vi "create channels for testing.vi"() -> (0 "2d names":string[][](array[string]), 1 "1d names":string[](array[string]), 2 "2d channels":refnum<class "Profibus channel.lvclass">[][](array[class]), 3 "1d channels":refnum<class "Profibus channel.lvclass">[](array[class]))   [LabVIEW 2013, in "Profibus Module tests.lvlib"]
uses:
  Profibus Module tests.lvlib
  channel/Profibus channel.lvclass
  <vilib>/NI/Tag Bus Module Framework/channel/channel classification.ctl
  configuration/Profibus Module configuration.lvclass
  <vilib>/NI/Tag Bus/tag/tag descriptor.lvclass/tag descriptor.ctl
  <vilib>/NI/Tag Bus Module Framework/channel/TBM channel.lvclass/TBM channel.ctl
  <vilib>/NI/Tag Bus/tag/write tag name.vi
  <vilib>/NI/Tag Bus/tag/write data type.vi
  <vilib>/NI/Tag Bus Module Framework/channel/Write channel classification.vi
  <vilib>/NI/Tag Bus Module Framework/channel/TBM channel.lvclass
  <vilib>/NI/Configuration Framework/serializable configuration/NISE_CEF_serializable configuration.lvclass
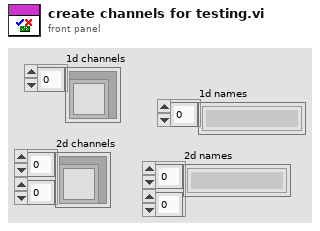
[diagram p1: front panel]
types:
  T1 = typedef "TBM channel.lvclass/channel classification.ctl" = enum16{"input data", "output data", "processing parameter", "processing result"}
  T2 = typedef "tag bus.lvlib/tag descriptor.lvclass/Data Type.ctl" = enum16{"Double", "Single", "I64", "I32", "I16", "I8", "U64", "U32", "U16", "U8", "Boolean", "String", "Array of Double", "Array of Single", "Array of I64", "Array of I32", "Array of I16", "Array of I8", "Array of U64", "Array of U32", "Array of U16", "Array of U8", "Array of Boolean", "Array of String"}
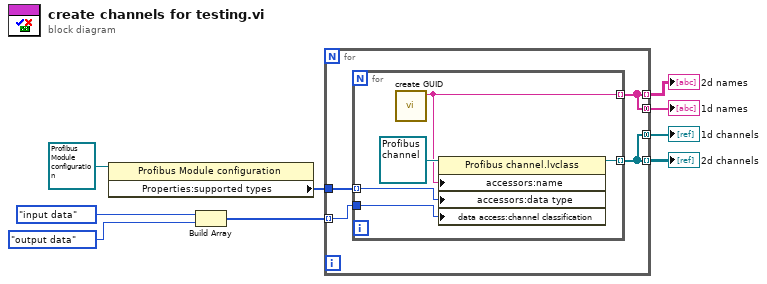
[diagram p0: block diagram]
diagram:
  n1 = property class="Profibus Module configuration"(reference=refnum<class "Profibus Module configuration.lvclass"> refnum ("tag bus configurable plugin module configuration")) -> ("Properties:supported types"=w9:T2[])  [unwired: 1 in, 2 out]
  n2 = Build Array(channel_classification."input data" ("channel classification"), channel_classification."output data" ("channel classification")) -> (w6:T1[])
  n3 = for {
    tunnel: w6 -> [w13] mode=indexing
    tunnel: [w11] -> w7 mode=concatenating
    tunnel: w9 -> [w12]
    tunnel: [w11] -> w3 mode=indexing
    tunnel: [w10] -> w1 mode=concatenating
    tunnel: [w10] -> w2 mode=indexing
    n4 = for {
      tunnel: w13 -> [w15]
      tunnel: [w17] -> w11 mode=indexing
      tunnel: w12 -> [w16] mode=indexing
      tunnel: [w14] -> w10 mode=indexing
      n5 = call <vilib>:"create GUID.vi"() -> ("uuid"=w14:string)  [unwired: 10 in, 1 out]
      n6 = property class="Profibus channel.lvclass"(reference=refnum<class "Profibus channel.lvclass"> refnum ("Profibus channel.lvclass"), "accessors:name"=w14, "accessors:data type"=w16, "data access:channel classification"=w15) -> (reference out=w17:refnum<class "Profibus channel.lvclass">)  [unwired: 1 in, 1 out]
    }
  }
  "1d channels" <- w7
  "2d channels" <- w3
  "2d names" <- w2
  "1d names" <- w1
